vi "m1m3_getSample_OuterLoopData.vi"(8 "error in (no error)":errorcluster, 11 "OuterLoopData_Ctl":T1) -> (0 "error out":errorcluster, 2 "function return":i32, 3 "OuterLoopData_Ctl out":T1)   [LabVIEW 2016, in "SALLV_m1m3.lvlib"]
doc: "int m1m3_shm_getSample_OuterLoopDataLV(m1m3_OuterLoopDataLV *OuterLoopData_Ctl );"
uses:
  SALLV_m1m3.lvlib
  DataTypes/OuterLoopData.ctl
  SALLV_m1m3.so
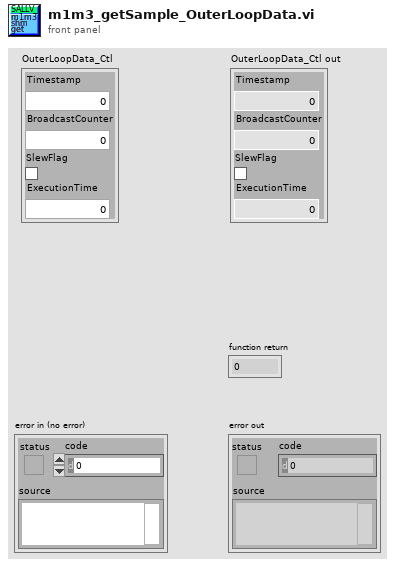
[diagram p1: front panel]
types:
  T1 = typedef "SALLV_m1m3.lvlib/OuterLoopData.ctl" = cluster{"Timestamp":dbl, "BroadcastCounter":i16, "SlewFlag":bool, "ExecutionTime":dbl}
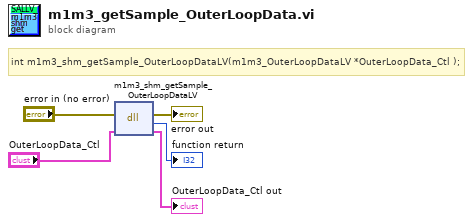
[diagram p0: block diagram]
diagram:
  # "int m1m3_shm_getSample_OuterLoopDataLV(m1m3_OuterLoopDataLV *OuterLoopData_Ctl );"
  n1 = dll-call lib="opt/CODE/SALLV_m1m3/SALLV_m1m3.*" fn="m1m3_shm_getSample_OuterLoopDataLV"(error in="error in (no error)", "OuterLoopData_Ctl"="OuterLoopData_Ctl") -> (error out=→"error out":errorcluster, →"function return":i32, "OuterLoopData_Ctl"=→"OuterLoopData_Ctl out":T1)  [unwired: 2 in, 1 out]
